vi "json_parser.vi"(8 "error in":errorcluster, 11 "JSON String":string) -> (0 "error out":errorcluster, 3 "JSON Tree Out Passthrough":variant)   [LabVIEW 2010]
uses:
  i3-json-1.0.0-10/JSON Parsing/Get Object Parameter Files/Get Object Parameter - Boolean.vi
  i3-json-1.0.0-10/JSON Parsing/Get Object Parameter Files/Get Object Parameter - String.vi
  i3-json-1.0.0-10/JSON Parsing/Get Object Parameter Files/Get Object Parameter - Array.vi
  i3-json-1.0.0-10/JSON Parsing/Get Array Value at Index Files/Get Array Value at Index - String.vi
  i3-json-1.0.0-10/i3-json.lvlib
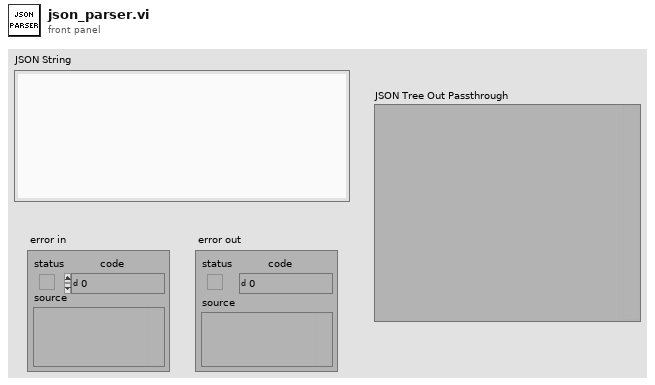
[diagram p1: front panel]
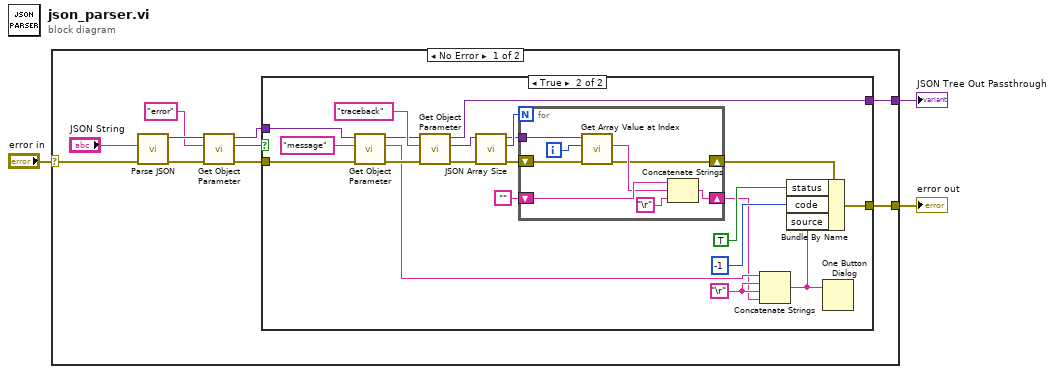
[diagram p0: block diagram]
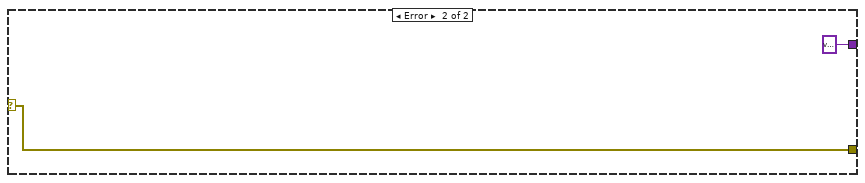
[diagram p3: hidden frame]
diagram:
  n1 = case shown="No Error" "error in" {
    selector: "error in" -> [w9 w46]
    tunnel: [w13 w46] -> w2
    tunnel: [w4 variant ("JSON Tree Out Passthrough 2")] -> w1
    frame No Error {
      n2 = call "Parse JSON.vi"("error in (no error)"=w9, "JSON String"="JSON String") -> ("error out"=w8:errorcluster, "JSON Tree"=w12:variant)  [unwired: 6 in, 2 out]
      n3 = call-poly "Get Object Parameter.vi"("error in (no error)"=w8, "Parameter Name"="error", "JSON Tree In (JSON Object)"=w12) -> ("error out"=w6:errorcluster, "Boolean Value"=w7:bool, "JSON Tree Out Passthrough"=w5:variant)  [unwired: 5 in, 1 out]
      n4 = case shown="True" w7 {
        tunnel: w6 -> [w14 w34]
        tunnel: [w14 w22] -> w13
        tunnel: w5 -> [w15 w35]
        tunnel: [w15 w30] -> w4
        frame False {
        }
        frame True {
          w20 = "\r"
          n5 = call-poly "Get Object Parameter.vi"("error in (no error)"=w34, "Parameter Name"="message", "JSON Tree In (JSON Object)"=w35) -> ("error out"=w32:errorcluster, "String Value"=w19:string, "JSON Tree Out Passthrough"=w31:variant)  [unwired: 5 in, 1 out]
          n6 = call-poly "Get Object Parameter.vi"("error in (no error)"=w32, "Parameter Name"="traceback", "JSON Tree In (JSON Object)"=w31) -> ("error out"=w26:errorcluster, "JSON Array"=w27:variant, "JSON Tree Out Passthrough"=w30:variant)  [unwired: 5 in, 1 out]
          n7 = call "JSON Array Size.vi"("error in (no error)"=w26, "JSON Tree In (JSON Array)"=w27) -> ("error out"=w25:errorcluster, "Array Size"=w29:i32, "JSON Tree Passthrough (JSON Array)"=w28:variant)  [unwired: 7 in]
          n8 = for {
            N: w29 -> [_]
            tunnel: w28 -> [w43]
            shift-right: [w41] -> w18
            shift-left: "" -> [w42]
            shift-right: [w38] -> w24
            shift-left: w25 -> [w39]
            i -> [w44]
            n9 = call-poly "Get Array Value at Index.vi"("error in (no error)"=w39, "Index"=w44, "JSON Tree In (JSON Array)"=w43) -> ("error out"=w38:errorcluster, "String Value"=w40:string)  [unwired: 5 in, 2 out]
            n10 = Concatenate Strings(w42, w40, "\r") -> (w41:string)
          }
          n11 = Concatenate Strings(w19, w20, w20, w18) -> (w17:string)
          n12 = Bundle By Name(cluster=w24, "status"=TRUE, "code"=-1, "source"=w17) -> (w22:errorcluster)
          n13 = One Button Dialog(message=w17) -> ()  [unwired: 1 in, 1 out]
        }
      }
    }
    frame Error {
    }
  }
  "error out" <- w2
  "JSON Tree Out Passthrough" <- w1
